vi "Check Execution Generic Execution.vi"() -> ()   [LabVIEW 2015]
panel:
  out "error out":errorcluster
  out "Cmd Text":string
  in  "TriggerIndex":i32
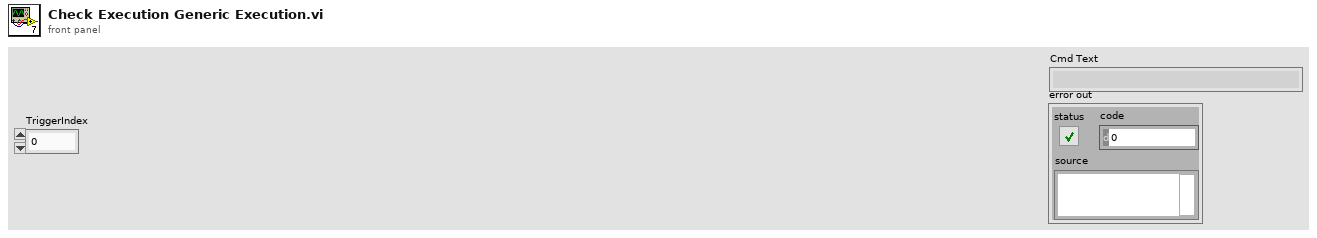
[diagram p1: front panel]
types:
  T1 = cluster{"Cmd Text":string, "MetaData":cluster{"Channel Name":string, "Index":i32, "Type":enum16{"List", "Channel"}, "List":string[], "ChannelFormat":string}[]}[]
  T2 = cluster{"Cmd Text":string, "MetaData":cluster{"Channel Name":string, "Index":i32, "Type":enum16{"List", "Channel"}, "List":string[], "ChannelFormat":string}[]}
  T3 = cluster{"Channel Name":string, "Index":i32, "Type":enum16{"List", "Channel"}, "List":string[], "ChannelFormat":string}[]
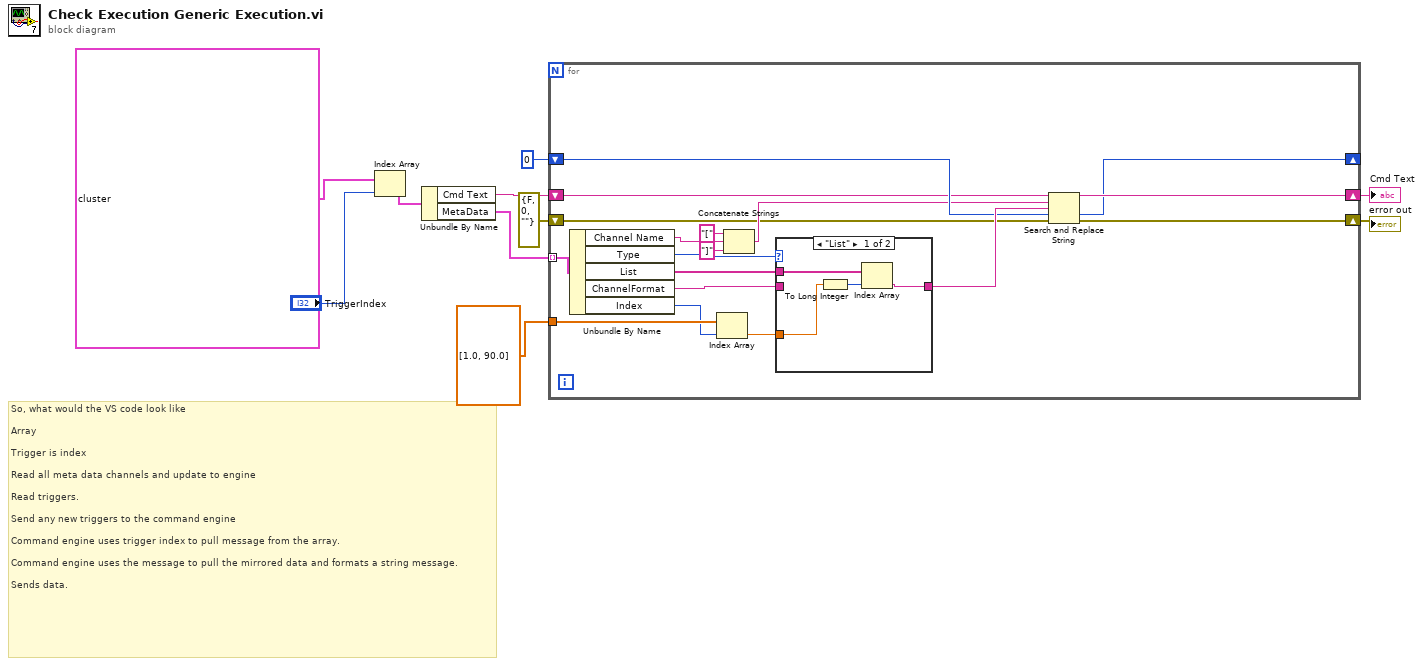
[diagram p0: block diagram]
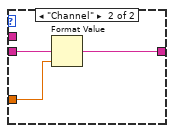
[diagram p2: hidden frame]
diagram:
  # "So, what would the VS code look like\n\nArray\n\nTrigger is index\n\nRead all meta data channels and update to engine\n\nRead triggers.\n\nSend any new triggers to the command engine\n\nCommand engine uses trigger index to pull message from the array.\n\nCommand engine uses the message to pull the mirrored data and formats a string message.\n\nSends data."
  n1 = Index Array(array=T1 [{"Cmd Text"="I Like:[People]:[Percentage]%", "MetaData"=[{"Channel Name"="People", "Index"=0, "Type"=enum."List", "List"=["Abby", "Noah", "Laura"], "ChannelFormat"=""}, {"Channel Name"="Percentage", "Index"=1, "Type"=enum."Channel", "List"=[], "ChannelFormat"="%.2f"}]}], index="TriggerIndex") -> (element=w8:T2)
  n2 = Unbundle By Name(w8) -> ("Cmd Text"=w7:string, "MetaData"=w6:T3)
  n3 = for {
    shift-right: [w15] -> w2
    shift-left: w7 -> [w16]
    shift-right: [w14] -> _
    shift-left: 0 -> [w17]
    tunnel: w6 -> [w28] mode=indexing
    tunnel: dbl[] [1.0, 90.0] -> [w23]
    shift-right: [w12] -> w1
    shift-left: errorcluster {"status"=FALSE, "code"=0, "source"=""} ("error out") -> [w11]
    n4 = Unbundle By Name(w28) -> ("Channel Name"=w27:string, "Type"=w24:enum16{"List", "Channel"}, "List"=w21:string[], "ChannelFormat"=w20:string, "Index"=w22:i32)
    n5 = Index Array(array=w23, index=w22) -> (element=w19:dbl)
    n6 = Concatenate Strings("[" ("string"), w27, "]" ("string")) -> (w13:string)
    n7 = case shown="\"List\"" w24 {
      tunnel: w21 -> [w32 _]
      tunnel: w20 -> [_ w35]
      tunnel: w19 -> [w31 w34]
      tunnel: [w29 w33] -> w18
      frame "List" {
        n8 = To Long Integer(number=w31) -> (32bit integer=w30:i32)
        n9 = Index Array(array=w32, index=w30) -> (element=w29:string)
      }
      frame "Channel" {
        n10 = Format Value(format string=w35, value (0)=w34) -> (output string=w33:string)  [unwired: 1 in]
      }
    }
    n11 = Search and Replace String(input string=w16, search string=w13, replace string=w18, offset=w17, error in=w11) -> (result string=w15:string, offset past replacement=w14:i32, error out=w12:errorcluster)  [unwired: 3 in, 1 out]
  }
  "Cmd Text" <- w2
  "error out" <- w1
